vi "UTF-8 to TXT.vi"(8 "error in":errorcluster, 10 "encoding (system default=-1)":i32, 11 "utf-8 text":string) -> (0 "error out":errorcluster, 3 "text":string)   [LabVIEW 2015]
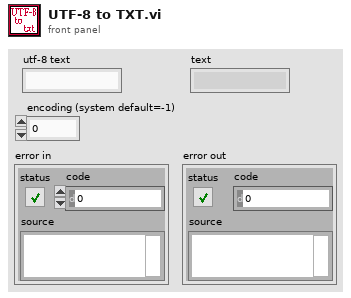
[diagram p1: front panel]
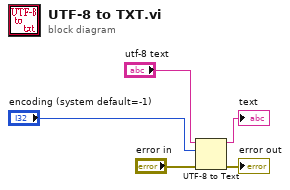
[diagram p0: block diagram]
diagram:
  n1 = UTF-8 to Text(8:"error in", 10:"encoding (system default=-1)", 11:"utf-8 text") -> (0:→"error out":errorcluster, 3:→"text":string)
